vi "GetRotorBarSidebandStep.vi"(9 "line frequency [Hz]":dbl, 10 "lower sidebands":T1, 11 "upper sidebands":T1) -> (3 "Rotor Sideband Step [Hz]":dbl)   [LabVIEW 2017, in "McsaAnalysisFunctions.lvlib"]
uses:
  <vilib>/addons/InsightCM/Utilities/Analysis/MCSA/McsaAnalysisFunctions.lvlib
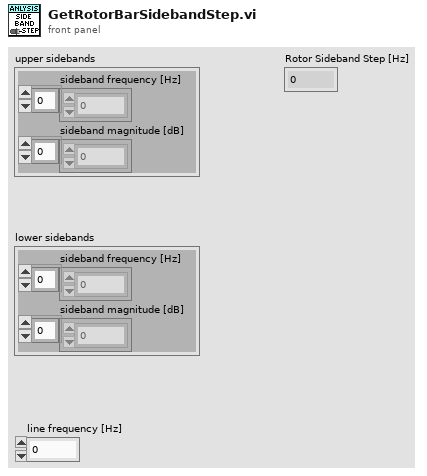
[diagram p1: front panel]
types:
  T1 = cluster{"sideband frequency [Hz]":dbl[], "sideband magnitude [dB]":dbl[]}
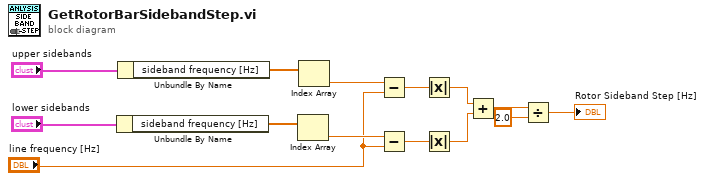
[diagram p0: block diagram]
diagram:
  n1 = Unbundle By Name("lower sidebands") -> ("sideband frequency [Hz]"=w11:dbl[])
  n2 = Unbundle By Name("upper sidebands") -> ("sideband frequency [Hz]"=w12:dbl[])
  n3 = Index Array(array=w11) -> (element=w9:dbl)  [unwired: 1 in]
  n4 = Index Array(array=w12) -> (element=w10:dbl)  [unwired: 1 in]
  n5 = Subtract(x=w10, y="line frequency [Hz]") -> (x-y=w8:dbl)
  n6 = Subtract(x=w9, y="line frequency [Hz]") -> (x-y=w7:dbl)
  n7 = Absolute Value(x=w8) -> (abs(x)=w6:dbl)
  n8 = Absolute Value(x=w7) -> (abs(x)=w5:dbl)
  n9 = Add(x=w6, y=w5) -> (x+y=w4:dbl)
  n10 = Divide(x=w4, y=2.0) -> (x/y=→"Rotor Sideband Step [Hz]":dbl)
